vi "Excel_OpenReference.vi"(5 "Template File Path":string="C:\\Users\\Candan\\Documents\\Sales Documents\\Gebze Customers\\Tubitak\\UME\\Guc Lab\\Ozlem Yilmaz\\TestStand Projesi\\14 Agustos 2015\\LVFiles\\Support\\Format_Table.xltx", 7 "File Visible ?":bool=TRUE, 8 "error in (no error)":errorcluster) -> (0 "error out":errorcluster, 1 "Sheets Reference Out":refnum<k7>, 2 "Workbook Reference Out":refnum<k7>, 3 "Excel Application Reference Out":refnum<k7>)   [LabVIEW 2014]
doc: "This VI demonstrates the use of ActiveX to write a table into a Microsoft Excel worksheet."
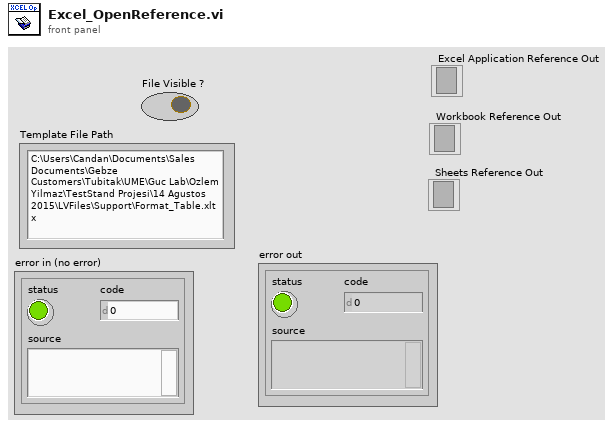
[diagram p1: front panel]
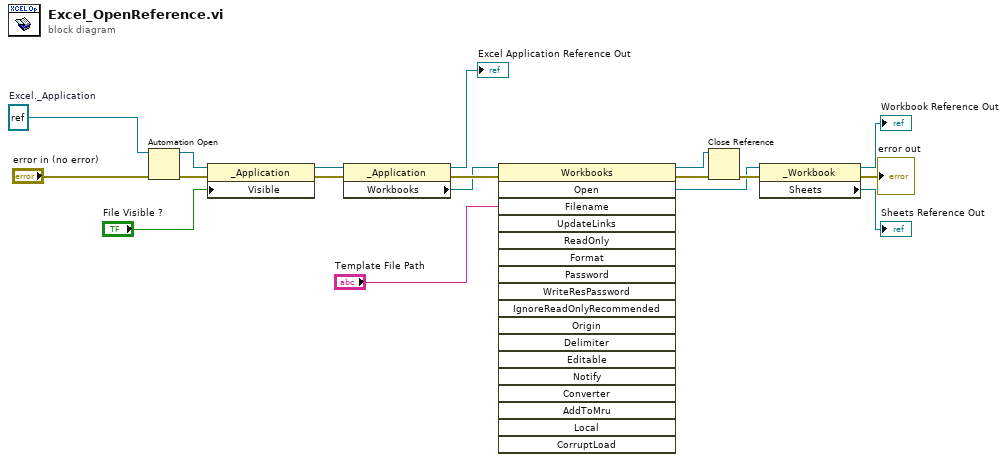
[diagram p0: block diagram]
diagram:
  w9 = refnum<k7> refnum  # Excel._Application
  n1 = Automation Open(error in (no error)="error in (no error)", Automation Refnum=w9) -> (Automation Refnum=w8:refnum<k7>, error out=w18:errorcluster)  [unwired: 2 out]
  n2 = property class="_Application"(reference=w8, error in=w18, "Visible"="File Visible ?") -> (reference out=w13:refnum<k7>, error out=w14:errorcluster)
  n3 = property class="_Application"(reference=w13, error in=w14) -> (reference out=→"Excel Application Reference Out":refnum<k7>, error out=w17:errorcluster, "Workbooks"=w11:refnum<k7>)
  n4 = invoke class="Workbooks" method="Open"(reference=w11, error in=w17, "Filename"="Template File Path") -> (reference out=w15:refnum<k7>, error out=w16:errorcluster, "Open"=w10:refnum<k7>)  [unwired: 15 in, 15 out]
  n5 = Close Reference(reference=w15, error in (no error)=w16) -> (error out=w12:errorcluster)
  n6 = property class="_Workbook"(reference=w10, error in=w12) -> (reference out=→"Workbook Reference Out":refnum<k7>, error out=→"error out":errorcluster, "Sheets"=→"Sheets Reference Out":refnum<k7>)
